vi "Estrai MD Contigui.vi"(10 "M REAL LETTURE":cluster{"MD":i16, "Descrizione":string}[](array[cluster])) -> (1 "Number MD":i32[](array[numeric]), 2 "ArrayMD":i32[](array[numeric]))   [LabVIEW 2019]
panel:
  out "x = y?":bool
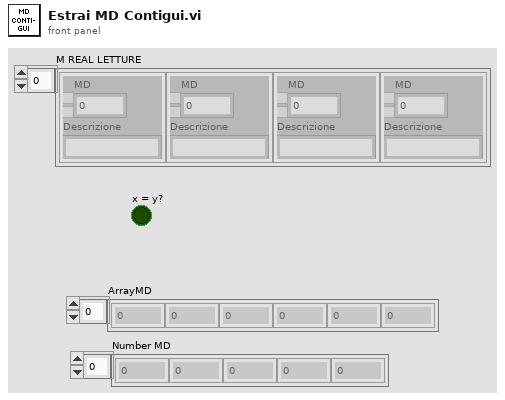
[diagram p1: front panel]
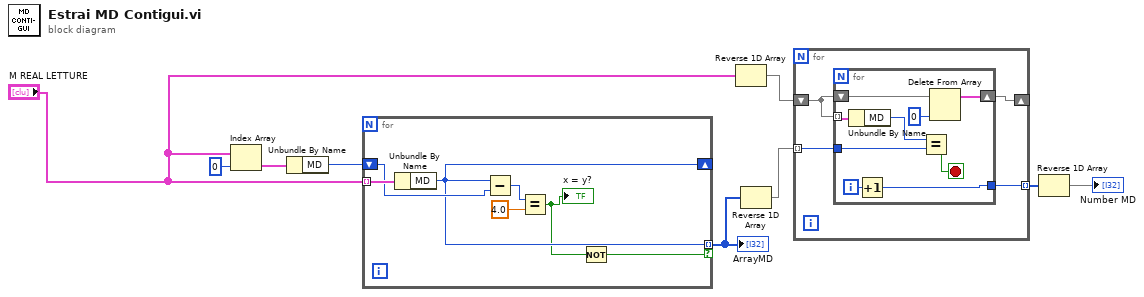
[diagram p0: block diagram]
diagram:
  n1 = Index Array(array="M REAL LETTURE", index=0) -> (element=w8:cluster{"MD":i16, "Descrizione":string})
  n2 = Unbundle By Name(w8) -> ("MD"=w7:i16)
  n3 = for {
    tunnel: "M REAL LETTURE" -> [w16] mode=indexing
    shift-right: [w12] -> _
    shift-left: w7 -> [w15]
    tunnel: [w12] -> w6 mode=indexing if=w11
    n4 = Unbundle By Name(w16) -> ("MD"=w12:i16)
    n5 = Subtract(x=w12, y=w15) -> (x-y=w14:i16)
    n6 = Equal?(x=w14, y=4.0) -> (x = y?=w10:bool)
    "x = y?" <- w10
    n7 = Not(x=w10) -> (.not. x?=w11:bool)
  }
  "ArrayMD" <- w6
  n8 = Reverse 1D Array(array="M REAL LETTURE") -> (reversed array=w4:cluster{"MD":i16, "Descrizione":string}[])
  n9 = Reverse 1D Array(array=w6) -> (reversed array=w5:i16[])
  n10 = for {
    tunnel: w5 -> [w20] mode=indexing
    shift-right: [w18] -> _
    shift-left: w4 -> [w19]
    tunnel: [w17] -> w3 mode=indexing
    n11 = for {
      tunnel: w19 -> [w29] mode=indexing
      tunnel: w20 -> [w27]
      shift-right: [w23] -> w18
      shift-left: w19 -> [w25]
      tunnel: [w21] -> w17
      i -> [w22]
      stop <- w26 stop-if-true
      n12 = Unbundle By Name(w29) -> ("MD"=w28:i16)
      n13 = Increment(x=w22) -> (x+1=w21:i32)
      n14 = Equal?(x=w28, y=w27) -> (x = y?=w26:bool)
      n15 = Delete From Array(array=w25, index=0) -> (array with subset deleted=w23:cluster{"MD":i16, "Descrizione":string}[])  [unwired: 1 in, 1 out]
    }
  }
  n16 = Reverse 1D Array(array=w3) -> (reversed array=→"Number MD":i32[])
